vi "Global Stop Actions.vi"(7 "Command":T1=enum."Read", 8 "error in (no error)":errorcluster, 9 "Stop on Error?":bool, 10 "Stop?":bool, 11 "vi reference":T2) -> (0 "error out":errorcluster {"code" min=0 max=0}, 1 "Skipped?":bool, 2 "Latched Stop":bool)   [LabVIEW 2013, in "Control Addon Engine.lvlib" / "Stop FG.lvlib"]
uses:
  Stop FG.lvlib
  Stop Global Ref.ctl
  Stop Global Commands.ctl
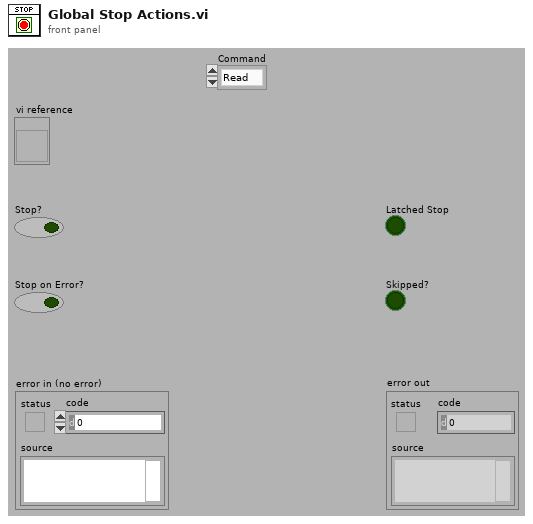
[diagram p1: front panel]
types:
  T1 = typedef "Control Addon Engine.lvlib/Stop FG.lvlib/Stop Global Commands.ctl" = enum16{"Write", "Read", "Reset"}
  T2 = typedef "Control Addon Engine.lvlib/Stop FG.lvlib/Stop Global Ref.ctl" = refnum<vi>
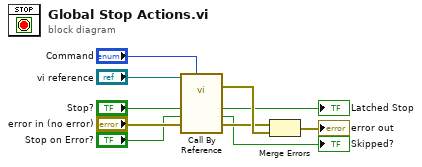
[diagram p0: block diagram]
diagram:
  n1 = call-by-ref "?"(reference="vi reference", "Command"="Command", "error in (no error)"="error in (no error)", "Stop on Error?"="Stop on Error?", "Stop?"="Stop?") -> (error out=w9:errorcluster, 0:"error out"=w6:errorcluster, "Skipped?"=→"Skipped?":bool, "Latched Stop"=→"Latched Stop":bool)  [unwired: 6 in, 1 out]
  n2 = Merge Errors(w6, w9) -> (→"error out":errorcluster)
